vi "RIGOL DS1000 Series Acquire Continuous Waveform.vi"() -> ()   [LabVIEW 2012]
doc: "This example shows how to use autosetup and acquire a waveform on a single channel."
uses:
  RIGOL DS1000 Series.lvlib
  Public/Data/Read (Single Waveform).vi
  <vilib>/measure/NI_MAPro.lvlib
  <vilib>/measure/madcrms.llb/Basic Averaged DC-RMS for 1 Chan.vi
panel:
  out "Power":waveform(dbl)(graph)
  out "Power":dbl
  in  "Channel (0: Channel 1) 3":u16(ring) items=["Channel 1", "Channel 2", "Channel 3", "Channel 4"]
  in  "Timeout (10000 ms) 3":u32=10000
  out "IRMS 2":dbl
  in  "Stop 3":bool
  out "Waveform Data 3":waveform(dbl)(graph)
  out "VRMS":dbl
  in  "Channel (0: Channel 1)":u16(ring) items=["Channel 1", "Channel 2", "Channel 3", "Channel 4"]
  in  "Stop":bool
  in  "Timeout (10000 ms)":u32=10000
  out "Waveform Data":waveform(dbl)(graph)
  in  "VISA resource name":refnum<visa-resource-name>
  # "(c) 2010-2012, RIGOL Technologies, Inc.  All Rights Reserved."
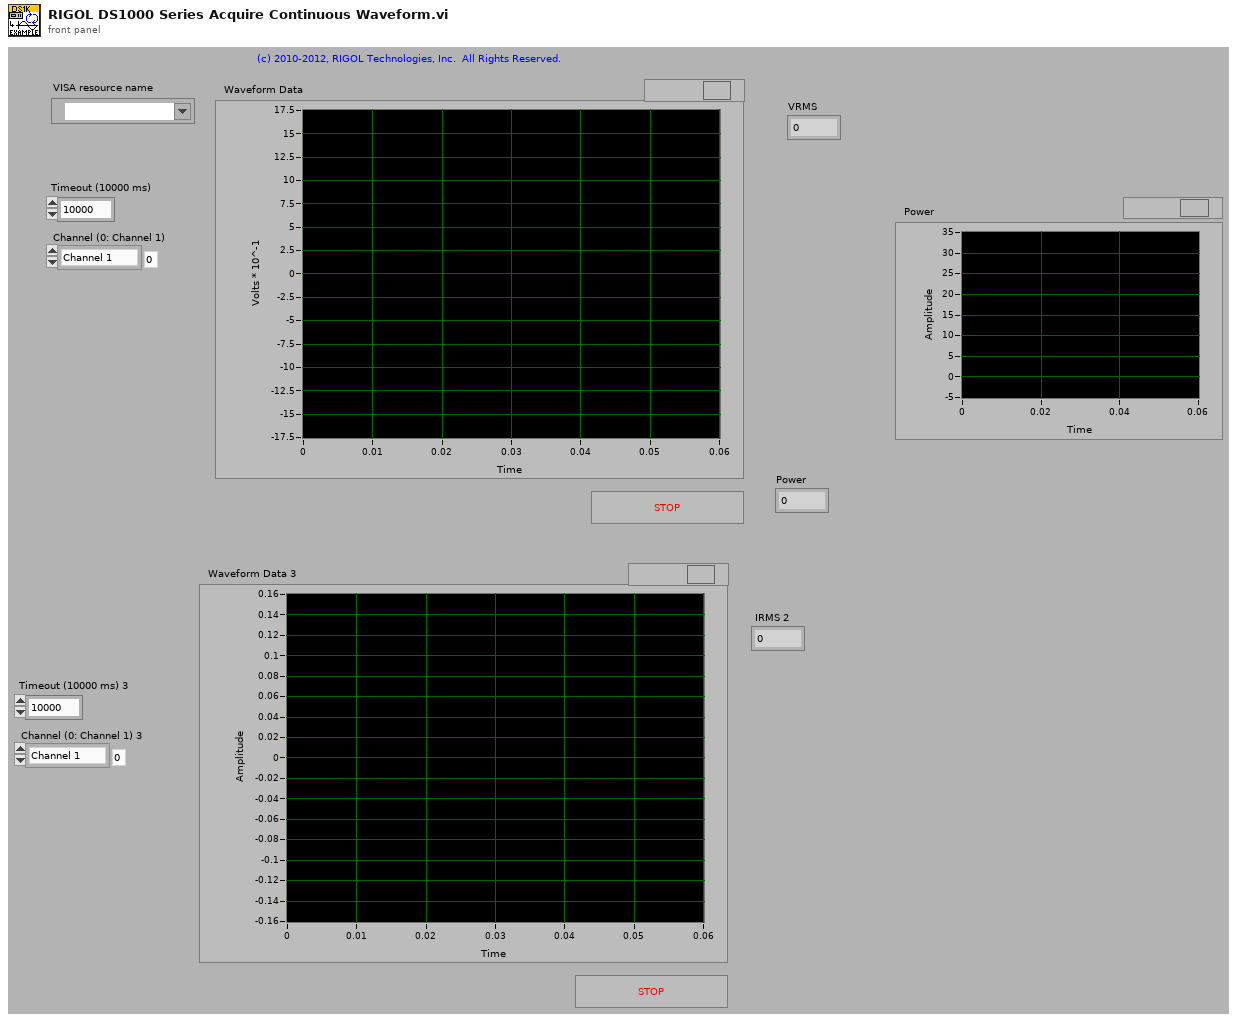
[diagram p1: front panel]
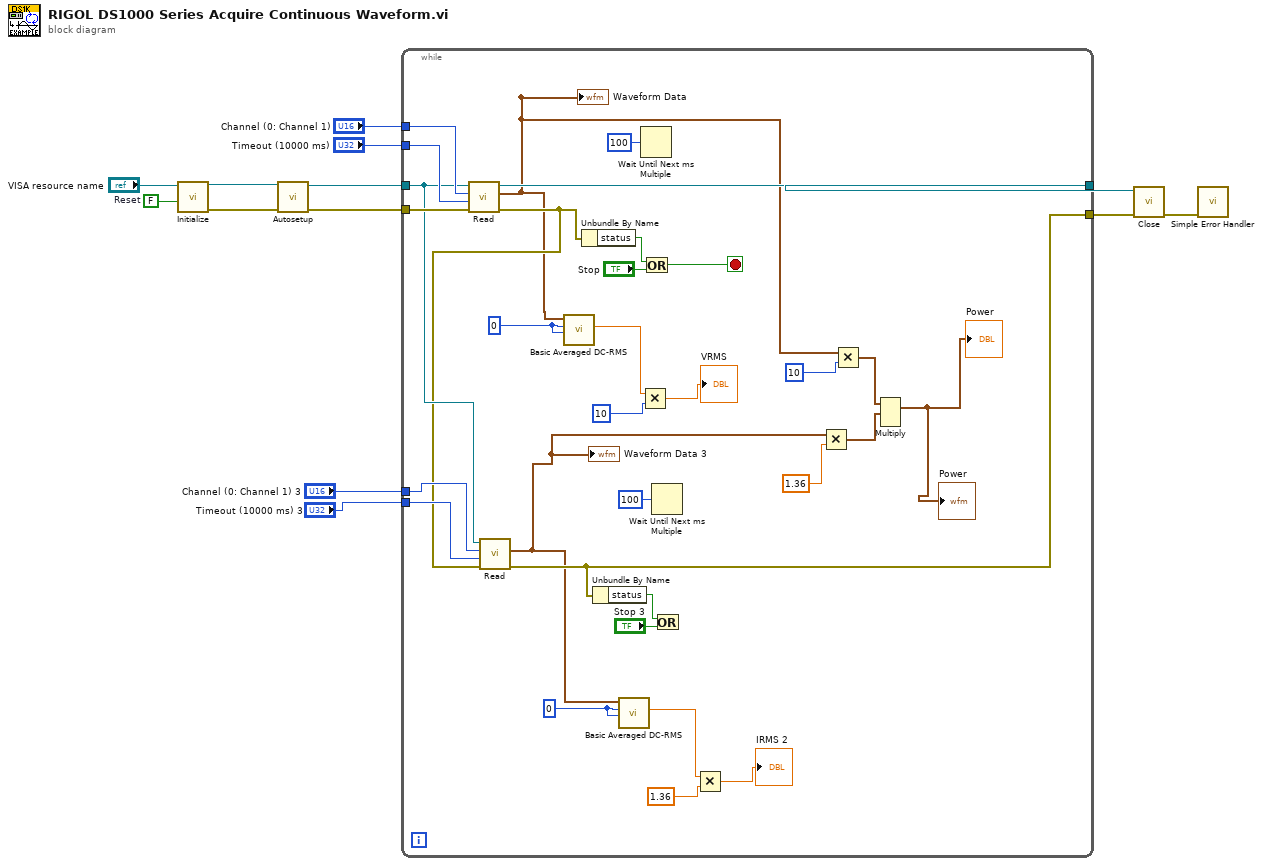
[diagram p0: block diagram]
diagram:
  w4 = FALSE  # Reset
  n1 = call "Initialize.vi"("Reset (True)"=w4, "VISA resource name"="VISA resource name") -> ("error out"=w9:errorcluster, "VISA resource name out"=w8:refnum<visa-resource-name>)  [unwired: 2 in, 6 out]
  n2 = call "Autosetup.vi"("error in (no error)"=w9, "VISA resource name"=w8) -> ("error out"=w6:errorcluster, "VISA resource name out"=w7:refnum<visa-resource-name>)  [unwired: 8 out]
  n3 = while {
    tunnel: w7 -> [w23]
    tunnel: w6 -> [w44]
    tunnel: [w43] -> w12
    tunnel: "Timeout (10000 ms)" -> [w37]
    tunnel: "Channel (0: Channel 1)" -> [w38]
    tunnel: "Channel (0: Channel 1) 3" -> [w25]
    tunnel: "Timeout (10000 ms) 3" -> [w24]
    tunnel: [w21] -> w1
    stop <- w41 stop-if-true
    w26 = 0
    w36 = 0
    n4 = call-poly "Read.vi"("error in (no error)"=w44, "Timeout (10000 ms)"=w37, "Channel (0: Channel 1)"=w38, "VISA resource name"=w23) -> ("error out"=w22:errorcluster, "Waveform Data"=w15:waveform(dbl), "VISA resource name out"=w43:refnum<visa-resource-name>)  [unwired: 5 out]
    "Waveform Data" <- w15
    n5 = call-poly "Read.vi"("error in (no error)"=w22, "Timeout (10000 ms)"=w24, "Channel (0: Channel 1)"=w25, "VISA resource name"=w23) -> ("error out"=w21:errorcluster, "Waveform Data"=w18:waveform(dbl))  [unwired: 6 out]
    "Waveform Data 3" <- w18
    n6 = call-poly <vilib>:"Basic Averaged DC-RMS.vi"("window"=w36, "averaging type"=w36, "signal in"=w15) -> ("RMS value"=w35:dbl)  [unwired: 5 in, 3 out]
    n7 = Unbundle By Name(w22) -> ("status"=w40:bool)
    n8 = Unbundle By Name(w21) -> ("status"=w31:bool)
    n9 = call-poly <vilib>:"Basic Averaged DC-RMS.vi"("window"=w26, "averaging type"=w26, "signal in"=w18) -> ("RMS value"=w27:dbl)  [unwired: 5 in, 3 out]
    n10 = Multiply(x=w35, y=10) -> (x*y=→"VRMS":dbl)
    n11 = Wait Until Next ms Multiple(millisecond multiple=u32 100) -> ()  [unwired: 1 out]
    n12 = Or(x=w40, y="Stop") -> (x .or. y?=w41:bool)
    n13 = Wait Until Next ms Multiple(millisecond multiple=u32 100) -> ()  [unwired: 1 out]
    n14 = Or(x=w31, y="Stop 3") -> ()  [unwired: 1 out]
    n15 = Multiply(x=w27, y=1.36) -> (x*y=→"IRMS 2":dbl)
    n16 = Multiply(x=w18, y=1.36) -> (x*y=w17:waveform(dbl))
    n17 = Multiply(x=w15, y=10) -> (x*y=w14:waveform(dbl))
    n18 = Multiply(1:w17, 2:w14) -> (0:→"Power" →"Power":waveform(dbl))  [unwired: 1 in, 1 out]
  }
  n19 = call "Close.vi"("error in (no error)"=w1, "VISA resource name"=w12) -> ("error out"=w13:errorcluster)  [unwired: 9 out]
  n20 = call <vilib>:"Simple Error Handler.vi"("error in (no error)"=w13) -> ()  [unwired: 1 in, 8 out]
